vi "MyQH Check Loop Error.vi"(9 "Fehler ignorieren":i32[](array[numeric]), 10 "Zu verarbeitende Feher":T1, 11 "Nachrichten-Queue":refnum<queue>) -> (2 "Fehler in Queue eingefügt?":bool, 3 "Nachrichten-Queue (Kopie)":refnum<queue>)   [LabVIEW 2014]
doc: "Fragt \"Zu verarbeitende Fehler\" ab und prüft, ob der Wert mit einem der Werte im Array \"Fehler ignorieren\" übereinstimmt. Wenn ja, wird nichts unternommen. Wenn nicht, ist eine Fehlernachricht mit den Fehlerdaten an die Schleife zur Nachrichtenverarbeitung zu übermitteln."
uses:
  Message Queue/Message Cluster.ctl
  Message Queue/Enqueue Message (Single).vi
  Message Queue/MyQH Message Queue.lvlib
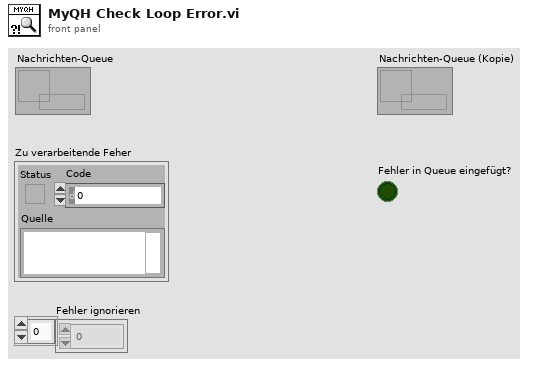
[diagram p1: front panel]
types:
  T1 = cluster{"Status":bool, "Code":i32, "Quelle":string}
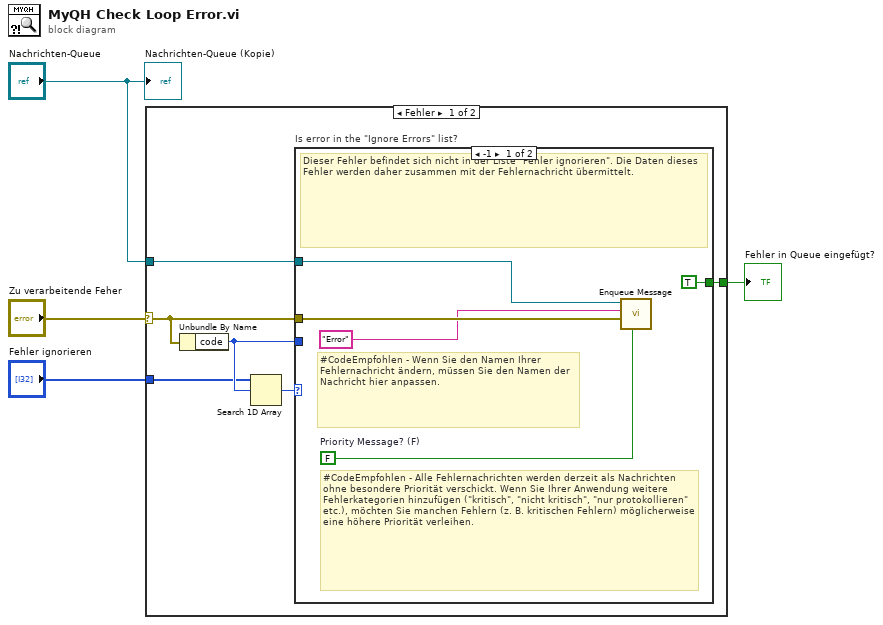
[diagram p0: block diagram]
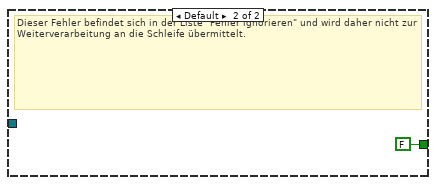
[diagram p2: hidden frame]
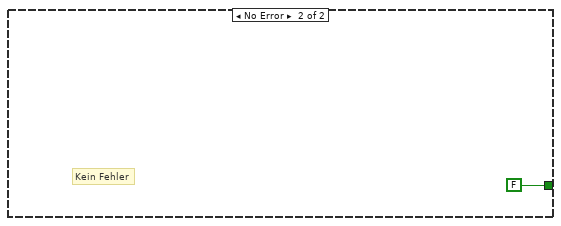
[diagram p3: hidden frame]
diagram:
  n1 = case shown="Fehler" "Zu verarbeitende Feher" {
    selector: "Zu verarbeitende Feher" -> [w7 _]
    tunnel: "Nachrichten-Queue" -> [w10 _]
    tunnel: "Fehler ignorieren" -> [w6 _]
    tunnel: [w5 FALSE] -> w1
    frame Error {
      n2 = Unbundle By Name(w7) -> ("code"=w8:i32)
      n3 = Search 1D Array(1D array=w6, element=w8) -> (index of element=w9:i32)  [unwired: 1 in]
      n4 = case "Is error in the \"Ignore Errors\" list?" shown="-1" w9 {
        tunnel: w7 -> [w13 _]
        tunnel: w10 -> [w15 _]
        tunnel: w8 -> [_ _]
        tunnel: [TRUE FALSE] -> w5
        frame -1 {
          w11 = FALSE  # Priority Message? (F)
          # "#CodeEmpfohlen - Alle Fehlernachrichten werden derzeit als Nachrichten ohne besondere Priorität verschickt. Wenn Sie Ihrer Anwendung weitere Fehlerkategorien hinzufügen (\"kritisch\", \"nicht kritisch\", \"nur protokollieren\" etc.), möchten Sie manchen Fehlern (z. B. kritischen Fehlern) möglicherweise eine höhere Priorität verleihen."
          # "#CodeEmpfohlen - Wenn Sie den Namen Ihrer Fehlernachricht ändern, müssen Sie den Namen der Nachricht hier anpassen."
          # "Dieser Fehler befindet sich nicht in der Liste \"Fehler ignorieren\". Die Daten dieses Fehler werden daher zusammen mit der Fehlernachricht übermittelt."
          n5 = call-poly "Enqueue Message.vi"("Nachricht mit Priorität? (F)"=w11, "Nachrichtendaten"=w13, "Nachricht"="Error" ("Message"), "Nachrichten-Queue"=w15) -> ()  [unwired: 6 in, 2 out]
        }
        frame Default {
          # "Dieser Fehler befindet sich in der Liste \"Fehler ignorieren\" und wird daher nicht zur Weiterverarbeitung an die Schleife übermittelt."
        }
      }
    }
    frame No Error {
      # "Kein Fehler"
    }
  }
  "Fehler in Queue eingefügt?" <- w1
  "Nachrichten-Queue (Kopie)" <- "Nachrichten-Queue"
